vi "F Dwf Analog In Status Samples Valid.vi"(8 "error in (no error)":errorcluster, 10 "pcSamplesValid":i32, 11 "hdwf":i32) -> (0 "error out":errorcluster, 2 "pcSamplesValid out":i32, 3 "function return":i32)   [LabVIEW 2019, in "Olasdwf.lvlib"]
doc: "DWFAPI int FDwfAnalogInStatusSamplesValid(HDWF hdwf, int *pcSamplesValid);"
uses:
  Olasdwf.lvlib
  Windows/System32/dwf.dll
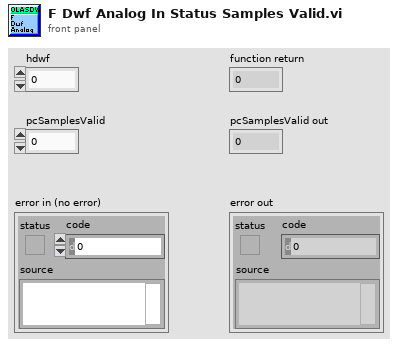
[diagram p1: front panel]
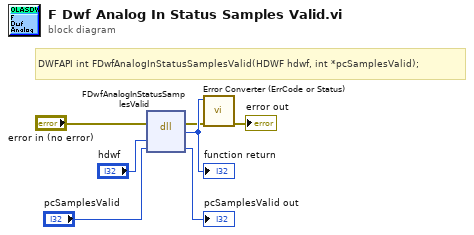
[diagram p0: block diagram]
diagram:
  # "DWFAPI int FDwfAnalogInStatusSamplesValid(HDWF hdwf, int *pcSamplesValid);"
  n1 = dll-call lib="C:/Windows/System32/dwf.*" fn="FDwfAnalogInStatusSamplesValid"(error in="error in (no error)", "hdwf"="hdwf", "pcSamplesValid"="pcSamplesValid") -> (error out=w2:errorcluster, w7:i32, "pcSamplesValid"=→"pcSamplesValid out":i32)  [unwired: 3 in, 1 out]
  "function return" <- w7
  n2 = call "Error Converter (ErrCode or Status).vi"("error in (no error)"=w2, "error code"=w7) -> ("error out"=→"error out":errorcluster)  [unwired: 9 in]
